vi "Write-Read Byte Array Demo.vi"() -> ()   [LabVIEW 2017]
panel:
  out "FT_Status":u32
  in  "Flow Control":u16(ring) items=["None"=0, "RTS-CTS"=256, "DTR-DSR"=512, "XOn-XOff"=1024]
  in  "Parity":u8(ring) items=["FT_PARITY_NONE", "FT_PARITY_ODD", "FT_PARITY_EVEN", "FT_PARITY_MARK", "FT_PARITY_SPACE"]
  in  "Stop Bits":u8(ring) items=["FT_STOP_BITS_1"=0, "FT_STOP_BITS_2"=2]
  in  "Word Length":u8(ring)=8 items=["FT_BITS_7"=7, "FT_BITS_8"=8]
  in  "Baud Rate":u64=9600
  out "Bytes Written":u32
  out "Device Description":string
  in  "Device Index":u32
  out "Read Buffer Out":u8[](array[numeric]) format="%x"
  out "Bytes Read":u32
  in  "Write Buffer":u8[](array[numeric]) format="%x"
  out "Bytes Waiting":u32
  # "Enter values in Write Buffer and run program.  \nWith a loop-back connector, the data is read back into the Read Buffer."
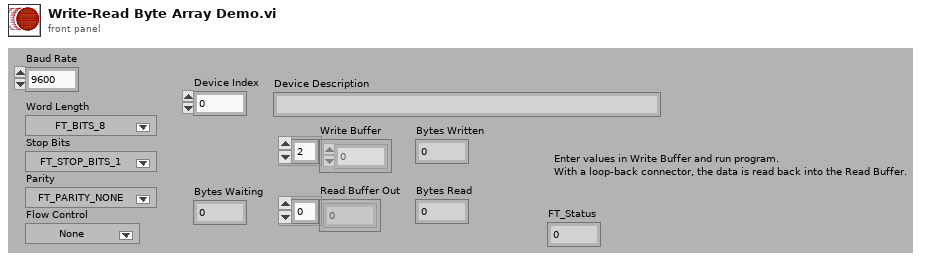
[diagram p1: front panel]
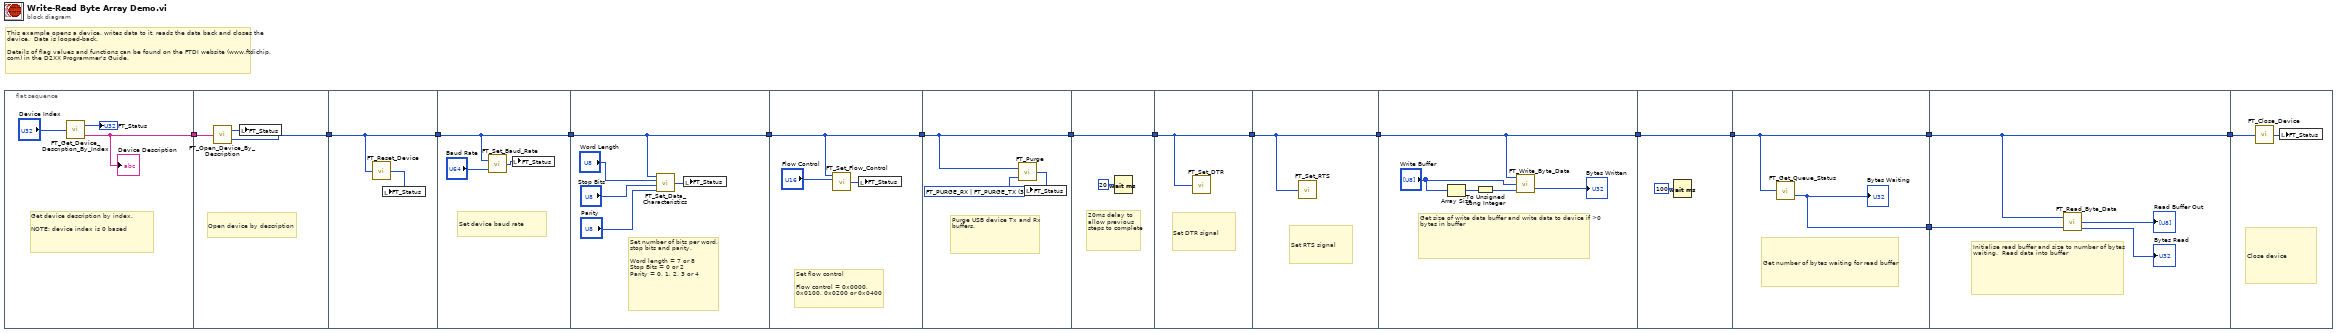
[diagram p0: block diagram]
diagram:
  # "This example opens a device, writes data to it, reads the data back and closes the device.  Data is looped-back.\n\nDetails of flag values and functions can be found on the FTDI website (www.ftdichip.com) in the D2XX Programmer's Guide."
  n1 = flat-sequence {
    tunnel: [w18] -> w11
    tunnel: [w19] -> w1
    tunnel: w11 -> [w21]
    tunnel: w1 -> [w23]
    tunnel: [w23] -> w9
    tunnel: w9 -> [w25]
    tunnel: [w25] -> w4
    tunnel: w4 -> [w31]
    tunnel: [w31] -> w15
    tunnel: w15 -> [w34]
    tunnel: [w34] -> w3
    tunnel: w3 -> [w37]
    tunnel: [w37] -> w2
    tunnel: [w38] -> w10
    tunnel: w2 -> [w38]
    tunnel: w10 -> [w40]
    tunnel: [w40] -> w8
    tunnel: w8 -> [w41]
    tunnel: [w41] -> w7
    tunnel: w7 -> [w46]
    tunnel: [w46] -> w6
    tunnel: w6 -> [w48]
    tunnel: [w48] -> w14
    tunnel: w14 -> [w50]
    tunnel: [w50] -> w13
    tunnel: [w49] -> w12
    tunnel: w13 -> [w53]
    tunnel: [w53] -> w5
    tunnel: w12 -> [w51]
    tunnel: w5 -> [w56]
    frame #0 {
      # "Get device description by index.\n\nNOTE: device index is 0 based"
      n2 = call "FT_Get_Device_Description_By_Index.vi"("Device Index"="Device Index") -> ("FT_Status"=→"FT_Status":u64, "Device Description"=w18:string)
      "Device Description" <- w18
    }
    frame #1 {
      # "Open device by description"
      n3 = call "FT_Open_Device_By_Description.vi"("Device Description"=w21) -> ("FT_Status"=w20:u64, "Handle"=w19:u64)
      n4 = local write "FT_Status"(w20) -> ()
    }
    frame #2 {
      n5 = call "FT_Reset_Device.vi"("Handle"=w23) -> ("FT_Status"=w22:u32)
      n6 = local write "FT_Status"(w22) -> ()
    }
    frame #3 {
      # "Set device baud rate"
      n7 = call "FT_Set_Baud_Rate.vi"("Baud Rate"="Baud Rate", "Handle"=w25) -> ("FT_Status"=w24:u64)
      n8 = local write "FT_Status"(w24) -> ()
    }
    frame #4 {
      # "Set number of bits per word, stop bits and parity.\n\nWord length = 7 or 8\nStop Bits = 0 or 2\nParity = 0, 1, 2, 3 or 4"
      n9 = call "FT_Set_Data_Characteristics.vi"("Parity"="Parity", "Stop Bits"="Stop Bits", "Word Length"="Word Length", "Handle"=w31) -> ("FT_Status"=w27:u32)
      n10 = local write "FT_Status"(w27) -> ()
    }
    frame #5 {
      # "Set flow control\n\nFlow control = 0x0000, 0x0100, 0x0200 or 0x0400"
      n11 = call "FT_Set_Flow_Control.vi"("Flow Control"="Flow Control", "Handle"=w34) -> ("FT_Status"=w32:u32)  [unwired: 2 in]
      n12 = local write "FT_Status"(w32) -> ()
    }
    frame #6 {
      w36 = u32 3 items=["FT_PURGE_RX"=1, "FT_PURGE_TX"=2, "FT_PURGE_RX | FT_PURGE_TX"=3] ("Purge Flags")
      # "Purge USB device Tx and Rx  buffers."
      n13 = call "FT_Purge.vi"("Purge Flags"=w36, "Handle"=w37) -> ("FT_Status"=w35:u32)
      n14 = local write "FT_Status"(w35) -> ()
    }
    frame #7 {
      # "20ms delay to allow previous steps to complete"
      n15 = Wait (ms)(milliseconds to wait=u32 20) -> ()  [unwired: 1 out]
    }
    frame #8 {
      # "Set DTR signal"
      n16 = call "FT_Set_DTR.vi"("Handle"=w40) -> ()  [unwired: 1 out]
    }
    frame #9 {
      # "Set RTS signal"
      n17 = call "FT_Set_RTS.vi"("Handle"=w41) -> ()  [unwired: 1 out]
    }
    frame #10 {
      # "Get size of write data buffer and write data to device if >0 bytes in buffer"
      n18 = Array Size(array="Write Buffer") -> (size(s)=w42:i32)
      n19 = To Unsigned Long Integer(number=w42) -> (unsigned 32bit integer=w43:u32)
      n20 = call "FT_Write_Byte_Data.vi"("Bytes To Write"=w43, "Buffer"="Write Buffer", "Handle"=w46) -> ("Bytes Written"=→"Bytes Written":u32)  [unwired: 1 out]
    }
    frame #11 {
      n21 = Wait (ms)(milliseconds to wait=u32 100) -> ()  [unwired: 1 out]
    }
    frame #12 {
      # "Get number of bytes waiting for read buffer"
      n22 = call "FT_Get_Queue_Status.vi"("Handle"=w50) -> ("Bytes Waiting"=w49:u32)  [unwired: 1 out]
      "Bytes Waiting" <- w49
    }
    frame #13 {
      # "Initialise read buffer and size to number of bytes waiting.  Read data into buffer"
      n23 = call "FT_Read_Byte_Data.vi"("Handle"=w53, "Bytes To Read"=w51) -> ("Read Data"=→"Read Buffer Out":u8[], "Bytes Read"=→"Bytes Read":u32)  [unwired: 1 out]
    }
    frame #14 {
      # "Close device"
      n24 = call "FT_Close_Device.vi"("Handle"=w56) -> ("FT_Status"=w55:u64)
      n25 = local write "FT_Status"(w55) -> ()
    }
  }
